vi "FT image and PID feedback (SubVI).vi"(0 "manual set amp.":dbl, 1 "PID gains":T1={"proportional gain (Kc)"=0.1, "integral time (Ti, min)"=1.0, "derivative time (Td, min)"=0.0} {"derivative time (Td, min)" format="%.3f"; "integral time (Ti, min)" format="%.3f"; "proportional gain (Kc)" format="%.3f"}, 2 "manual set?":bool, 3 "Polyfit Coeff. \n(amp. to position)":dbl[](array[numeric]), 5 "Image with Extract":T3, 7 "set amp.":dbl, 9 "select fre.":i32, 12 "T=feedback; F=not":bool, 14 "output range":cluster{"output high":dbl, "output low":dbl}={"output high"=11.0, "output low"=9.0} {"output low" format="%.2f"; "output high" format="%.2f"}, 15 "ms to wait for PID":u32=50) -> (4 "z position before move\nor no feedback=z drift (um)":dbl, 6 "z position of PID target (um)":dbl, 8 "current amp.":dbl, 10 "z position after moved (um)":dbl, 13 "relative seconds":dbl format="%_19f")   [LabVIEW 2014]
uses:
  <vilib>/vision/Image Controls.llb/IMAQ Image.ctl
  <vilib>/Analysis/baseanly.llb/Mean (DBL).vi
  <vilib>/Analysis/NI_AALBase.lvlib
panel:
  in  "# of avg. loop":i32=20
  in  "milliseconds to wait 2":u32=10
  in  "milliseconds to wait":u32=10
  in  "BCG Values":T2={"Brightness"=200.0, "Contrast"=50.0, "Gamma"=1.0}
  in  "adjust?":bool
  out "Number of Matches (Shape Detection 1)":i32
  out "Circles (Shape Detection 1)":T4(array[cluster]) {"Position"."Y" format="%.2f"; "Position"."X" format="%.2f"}
  in  "ROI Descriptor (Shape Detection 1)":T5={"Global Rectangle"=[6, 17, 113, 117], "Contours"=[{"ID"=enum."External", "Type"=3, "Coordinates"=[6, 17, 113, 117]}]} {"Contours"."Type" items=["No Selection", "Point", "Line", "Rectangle", "Oval", "Polygon", "Freehand Region", "Annulus", "Unused2", "Unused3", "Broken Line", "Freehand Line", "Rotated Rectangle"]}
  in  "Curve Parameters (Shape Detection 1)":T6={"Extraction Mode"=0, "Edge Threshold"=11, "Edge Filter Size"=1, "Min Length"=1, "Row Search Step Size"=1, "Col Search Step Size"=1, "Max Endpoint Gap"=1, "Closed"=FALSE, "Subpixel"=FALSE} {"Extraction Mode" items=["Normal", "Uniform Regions"]; "Edge Filter Size" items=["Fine", "Normal"]}
  in  "Minimum match score (Shape Detection 1)":dbl=800.0
  in  "Match Options (Shape Detection 1)":T7={"Rotation"=TRUE, "Scale"=FALSE, "Occlusion"=FALSE, "Range Settings"=[{"Match Constraints"=0, "Min"=0.0, "Max"=360.0}]} {"Range Settings"."Match Constraints" items=["Rotation Angle (degrees)", "Scale Factor (%)", "Occlusion (%)"]}
  in  "Remaining Inputs":T8={"Circle Descriptor (Shape Detection 1)"={"Min Radius"=3.0, "Max Radius"=500.0}, "Y Scale.Mapping Mode (Line Profile 1)"=0}
  out "Pixels Line (U8)":u8[](array[numeric])
  out "Waveform Graph":u8[](graph)
  out "Waveform Graph 2":dbl[](graph)
  out "# found":i32
  out "Image dup":T3(plugin-control)
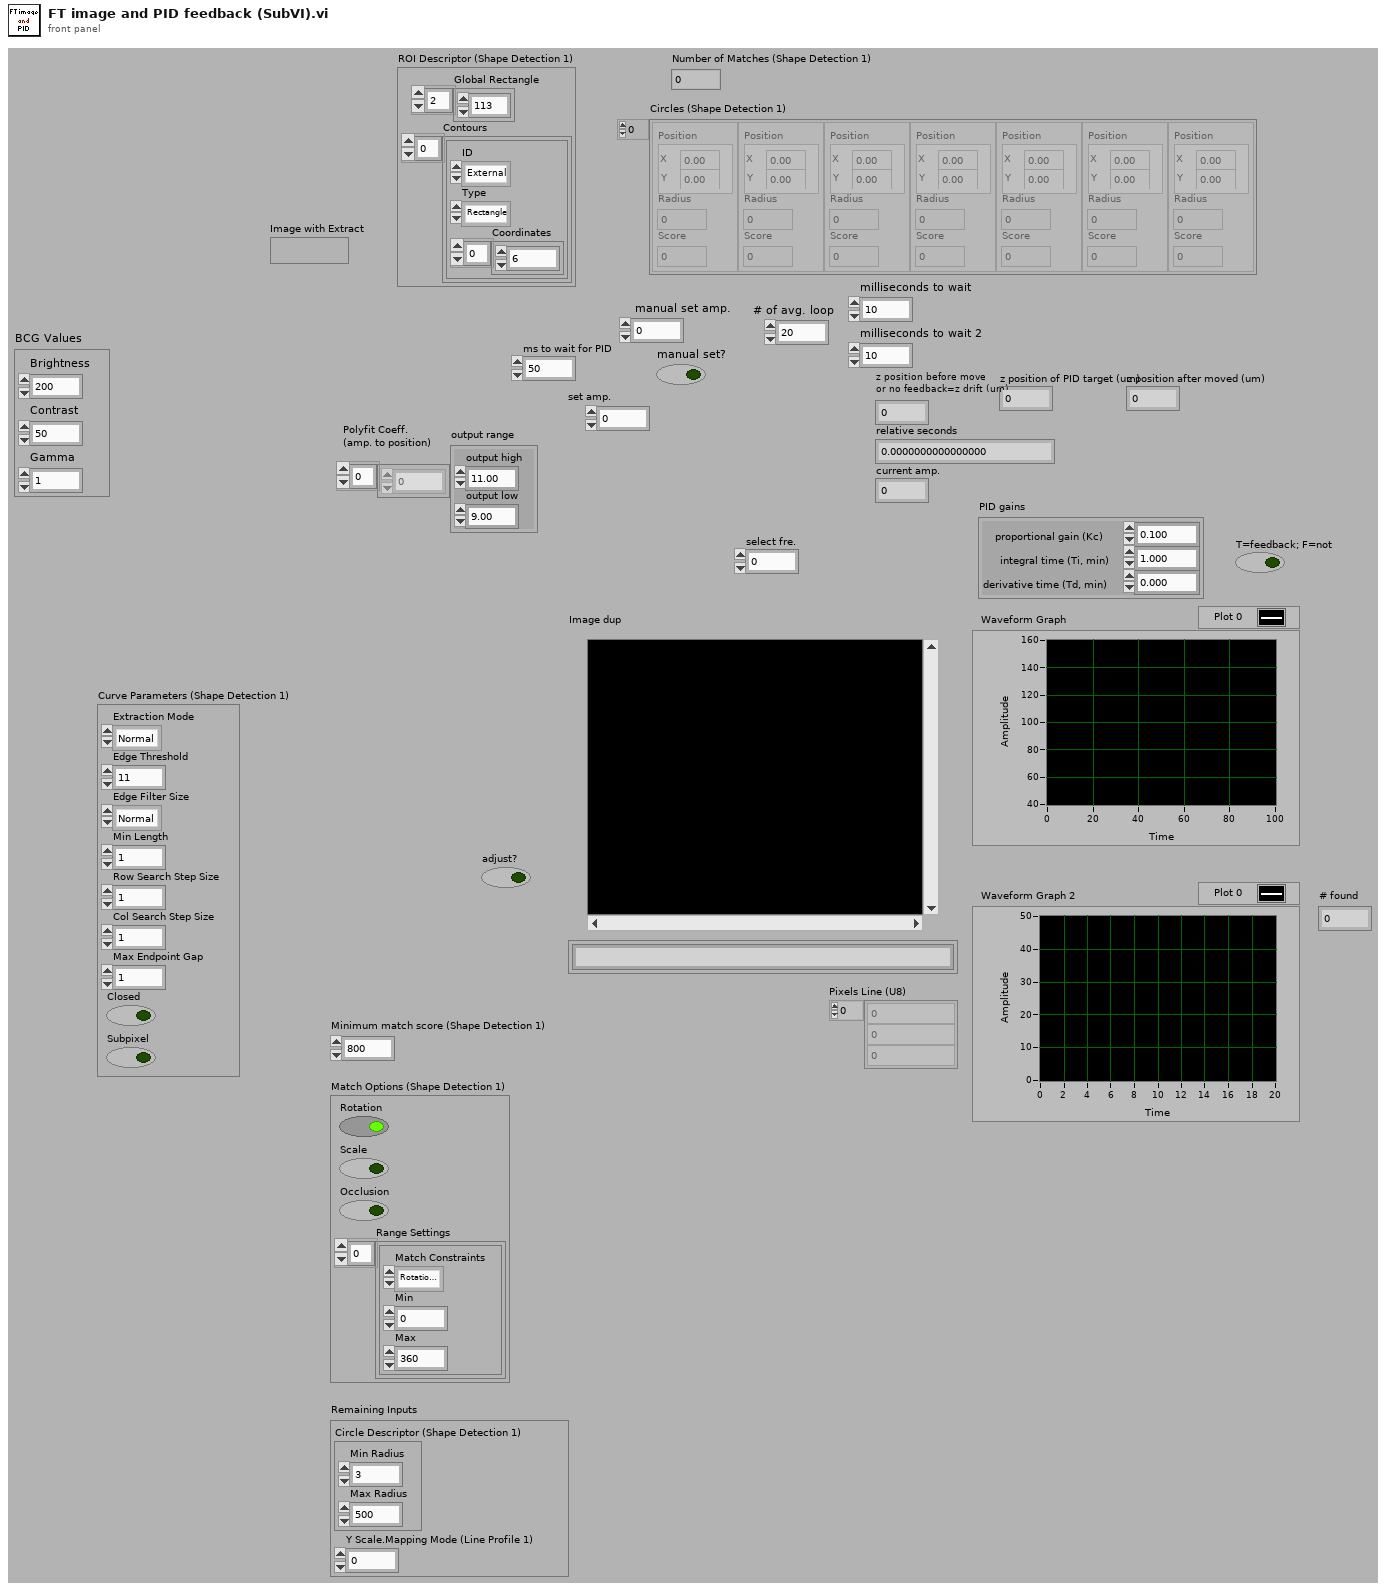
[diagram p1: front panel]
types:
  T1 = cluster{"proportional gain (Kc)":dbl, "integral time (Ti, min)":dbl, "derivative time (Td, min)":dbl}
  T2 = cluster{"Brightness":sgl, "Contrast":sgl, "Gamma":sgl}
  T3 = typedef "IMAQ Image.ctl" = refnum<image>
  T4 = cluster{"Position":cluster{"X":sgl, "Y":sgl}, "Radius":dbl, "Score":dbl}[]
  T5 = cluster{"Global Rectangle":i32[], "Contours":cluster{"ID":enum32{"External", "Internal"}, "Type":u32, "Coordinates":i32[]}[]}
  T6 = cluster{"Extraction Mode":u32, "Edge Threshold":i32, "Edge Filter Size":u32, "Min Length":i32, "Row Search Step Size":i32, "Col Search Step Size":i32, "Max Endpoint Gap":i32, "Closed":bool, "Subpixel":bool}
  T7 = cluster{"Rotation":bool, "Scale":bool, "Occlusion":bool, "Range Settings":cluster{"Match Constraints":u32, "Min":dbl, "Max":dbl}[]}
  T8 = cluster{"Circle Descriptor (Shape Detection 1)":cluster{"Min Radius":dbl, "Max Radius":dbl}, "Y Scale.Mapping Mode (Line Profile 1)":u8}
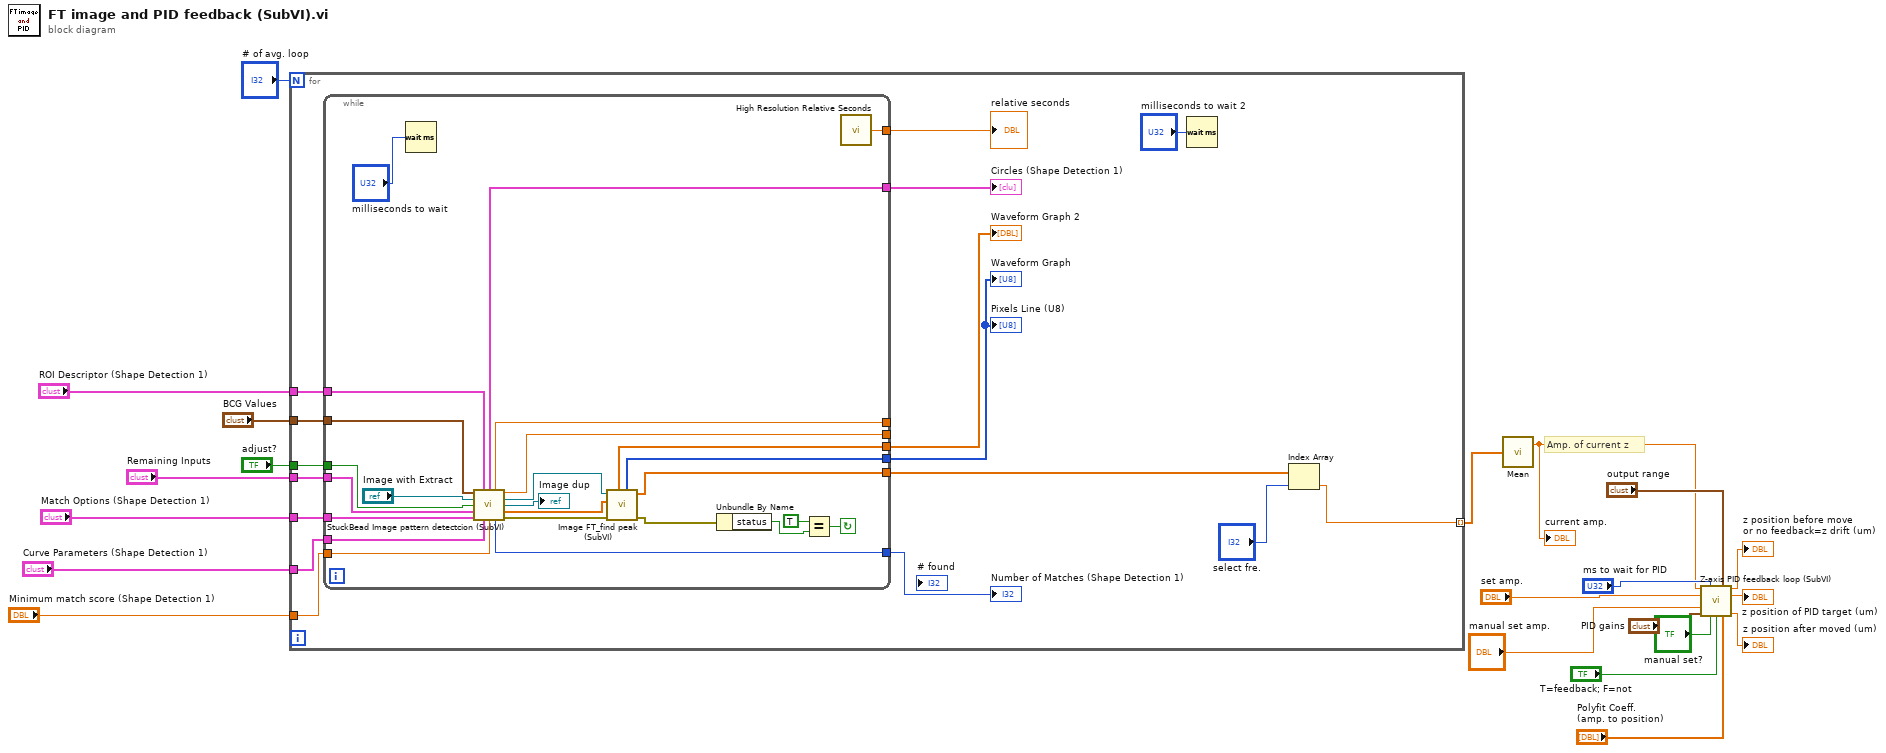
[diagram p0: block diagram]
diagram:
  # "Amp. of current z"
  n1 = for {
    N: "# of avg. loop" -> [_]
    tunnel: "ROI Descriptor (Shape Detection 1)" -> [w37]
    tunnel: "Minimum match score (Shape Detection 1)" -> [w36]
    tunnel: "Curve Parameters (Shape Detection 1)" -> [w35]
    tunnel: "Match Options (Shape Detection 1)" -> [w32]
    tunnel: "Remaining Inputs" -> [w31]
    tunnel: "adjust?" -> [w30]
    tunnel: "BCG Values" -> [w29]
    tunnel: [w24] -> w5 mode=indexing
    n2 = while {
      tunnel: w37 -> [w62]
      tunnel: w36 -> [w61]
      tunnel: w35 -> [w60]
      tunnel: [w59] -> w34
      tunnel: [w58] -> w33
      tunnel: w32 -> [w57]
      tunnel: w31 -> [w56]
      tunnel: w30 -> [w55]
      tunnel: w29 -> [w53]
      tunnel: [w48] -> w28
      tunnel: [w47] -> w27
      tunnel: [w46] -> _
      tunnel: [w45] -> _
      tunnel: [w42] -> w26
      tunnel: [w41] -> w25
      stop <- w43 continue-if-true
      n3 = Wait (ms)(milliseconds to wait="milliseconds to wait") -> ()  [unwired: 1 out]
      n4 = call "StuckBead Image pattern detectcion (SubVI).vi"("BCG Values"=w53, "ROI Descriptor (Shape Detection 1)"=w62, "Refnum in"="Image with Extract", "adjust?"=w55, "Remaining Inputs"=w56, "Match Options (Shape Detection 1)"=w57, "Curve Parameters (Shape Detection 1)"=w60, "Minimum match score (Shape Detection 1)"=w61) -> ("Circles (Shape Detection 1)"=w59:T4, "X posiiton on image \n(pattern detection)"=w46:sgl, "Y posiiton on image \n(pattern detection)"=w45:sgl, "Refnum out"=w51:T3, "Image dup"=→"Image dup":T3, "Array"=w50:sgl[], "Number of Matches (Shape Detection 1)"=w58:i32, "error out"=w49:errorcluster)
      n5 = call "Image FT_find peak (SubVI).vi"("error in (no error)"=w49, "Array"=w50, "Refnum in"=w51) -> ("error out"=w40:errorcluster, "Power Spectrum"=w41:dbl[], "Pixels Line (U8)"=w48:u8[], "Waveform Graph 2"=w47:dbl[])  [unwired: 2 in, 3 out]
      n6 = Unbundle By Name(w40) -> ("status"=w39:bool)
      n7 = Equal?(x=TRUE ("status"), y=w39) -> (x = y?=w43:bool)
      n8 = call <vilib>:"High Resolution Relative Seconds.vi"() -> ("relative seconds"=w42:dbl)
    }
    "Number of Matches (Shape Detection 1)" <- w33
    "Circles (Shape Detection 1)" <- w34
    "Pixels Line (U8)" <- w28
    "Waveform Graph" <- w28
    "Waveform Graph 2" <- w27
    "relative seconds" <- w26
    n9 = Wait (ms)(milliseconds to wait="milliseconds to wait 2") -> ()  [unwired: 1 out]
    n10 = Index Array(array=w25, index="select fre.") -> (element=w24:dbl)
  }
  n11 = call-poly <vilib>:"Mean.vi"("X"=w5) -> ("mean"=w6:dbl)  [unwired: 1 out]
  "current amp." <- w6
  n12 = call "Z-axis PID feedback loop (SubVI).vi"("current amp."=w6, "ms to wait for PID"="ms to wait for PID", "output range"="output range", "set amp."="set amp.", "manual set amp."="manual set amp.", "PID gains"="PID gains", "manual set?"="manual set?", "T=feedback; F=not"="T=feedback; F=not", "Polyfit Coeff. \n(amp. to position)"="Polyfit Coeff. \n(amp. to position)") -> ("z position before move\nor no feedback=z drift (um)"=→"z position before move\nor no feedback=z drift (um)":dbl, "z position of PID target (um)"=→"z position of PID target (um)":dbl, "z position after moved (um)"=→"z position after moved (um)":dbl)  [unwired: 4 in]
